vi "Get Meta Data.vi"(7 "Unique ID":string, 8 "error in (no error)":errorcluster, 11 "Test Executive in":refnum<class "Test Executive.lvclass">) -> (0 "error out":errorcluster, 2 "Meta Data":string, 3 "Test Executive out":refnum<class "Test Executive.lvclass">)   [LabVIEW 2020, in "Test Executive.lvlib" / "Test Executive.lvclass"]
uses:
  <vilib>/gpm_packages/@cs/test-executive/Source/Test Executive/TestExecutive/Test Executive.lvclass
  <vilib>/gpm_packages/@cs/test-executive/Source/Test Executive/TestExecutive/Test Executive.lvclass/Test Executive.ctl
  <vilib>/gpm_packages/@cs/linked-list/Source/Linked List/Linked List Ref/Linked List Ref.lvclass
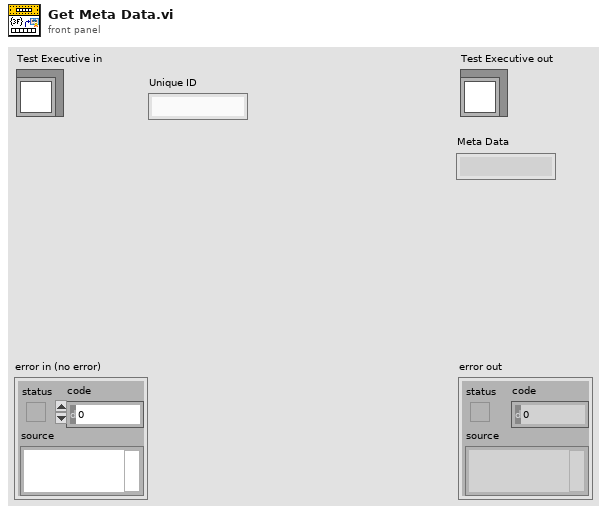
[diagram p1: front panel]
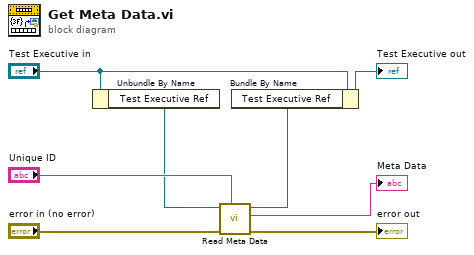
[diagram p0: block diagram]
diagram:
  n1 = Unbundle By Name("Test Executive in") -> ("Test Executive Ref"=w4:refnum<data-value>)
  n2 = call <vilib>:"Read Meta Data.vi"("Linked List ID"="Unique ID", "error in (no error)"="error in (no error)", "Linked List Ref"=w4) -> ("error out"=→"error out":errorcluster, "Meta Data"=→"Meta Data":string, "Linked List Ref out"=w1:refnum<data-value>)  [unwired: 5 in, 1 out]
  n3 = Bundle By Name(cluster="Test Executive in", "Test Executive Ref"=w1) -> (→"Test Executive out":refnum<class "Test Executive.lvclass">)
